vi "Initialize.vi"(8 "landscape?":bool, 9 "column":i16, 10 "row":i16, 11 "Component.lvclass in":refnum<class "Component.lvclass">) -> (3 "Component.lvclass out":refnum<class "Component.lvclass">)   [LabVIEW 2023, in "Component.lvclass"]
doc: "Initialize this component."
uses:
  Component.lvclass
  Component.lvclass/Component.ctl
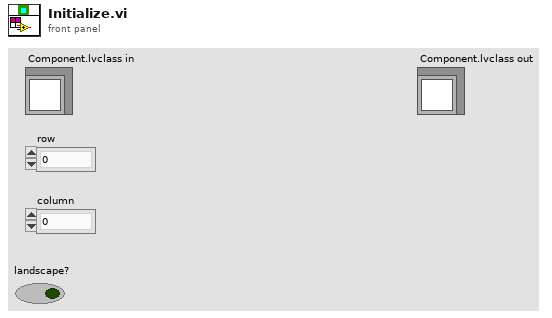
[diagram p1: front panel]
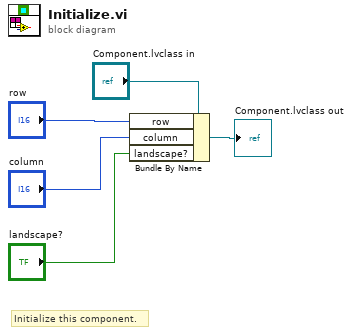
[diagram p0: block diagram]
diagram:
  # "Initialize this component."
  n1 = Bundle By Name(cluster="Component.lvclass in", "row"="row", "column"="column", "landscape?"="landscape?") -> (→"Component.lvclass out":refnum<class "Component.lvclass">)
